vi "Pigeon2Getters.vi"   [LabVIEW 2023]
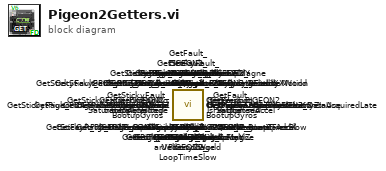
[diagram p0: block diagram]
diagram:
  n1 = call <vilib>:"GetStickyFault_PIGEON2_SaturatedGyros.vi"() -> ()  [unwired: 11 in, 1 out]
  n2 = call <vilib>:"GetFault_PIGEON2_SaturatedGyros.vi"() -> ()  [unwired: 11 in, 1 out]
  n3 = call <vilib>:"GetStickyFault_PIGEON2_SaturatedAccel.vi"() -> ()  [unwired: 11 in, 1 out]
  n4 = call <vilib>:"GetFault_PIGEON2_SaturatedAccel.vi"() -> ()  [unwired: 11 in, 1 out]
  n5 = call <vilib>:"GetStickyFault_PIGEON2_SaturatedMagne.vi"() -> ()  [unwired: 11 in, 1 out]
  n6 = call <vilib>:"GetFault_PIGEON2_SaturatedMagne.vi"() -> ()  [unwired: 11 in, 1 out]
  n7 = call <vilib>:"GetStickyFault_PIGEON2_LoopTimeSlow.vi"() -> ()  [unwired: 11 in, 1 out]
  n8 = call <vilib>:"GetFault_PIGEON2_LoopTimeSlow.vi"() -> ()  [unwired: 11 in, 1 out]
  n9 = call <vilib>:"GetStickyFault_PIGEON2_DataAcquiredLate.vi"() -> ()  [unwired: 11 in, 1 out]
  n10 = call <vilib>:"GetFault_PIGEON2_DataAcquiredLate.vi"() -> ()  [unwired: 11 in, 1 out]
  n11 = call <vilib>:"GetStickyFault_PIGEON2_BootIntoMotion.vi"() -> ()  [unwired: 11 in, 1 out]
  n12 = call <vilib>:"GetFault_PIGEON2_BootIntoMotion.vi"() -> ()  [unwired: 11 in, 1 out]
  n13 = call <vilib>:"GetStickyFault_PIGEON2_BootupMagne.vi"() -> ()  [unwired: 11 in, 1 out]
  n14 = call <vilib>:"GetFault_PIGEON2_BootupMagne.vi"() -> ()  [unwired: 11 in, 1 out]
  n15 = call <vilib>:"GetStickyFault_PIGEON2_BootupGyros.vi"() -> ()  [unwired: 11 in, 1 out]
  n16 = call <vilib>:"GetFault_PIGEON2_BootupGyros.vi"() -> ()  [unwired: 11 in, 1 out]
  n17 = call <vilib>:"GetStickyFault_PIGEON2_BootupAccel.vi"() -> ()  [unwired: 11 in, 1 out]
  n18 = call <vilib>:"GetFault_PIGEON2_BootupAccel.vi"() -> ()  [unwired: 11 in, 1 out]
  n19 = call <vilib>:"GetStickyFault_UnlicensedFeatureInUse.vi"() -> ()  [unwired: 11 in, 1 out]
  n20 = call <vilib>:"GetFault_UnlicensedFeatureInUse.vi"() -> ()  [unwired: 11 in, 1 out]
  n21 = call <vilib>:"GetStickyFault_BootDuringEnable.vi"() -> ()  [unwired: 11 in, 1 out]
  n22 = call <vilib>:"GetFault_BootDuringEnable.vi"() -> ()  [unwired: 11 in, 1 out]
  n23 = call <vilib>:"GetStickyFault_Undervoltage.vi"() -> ()  [unwired: 11 in, 1 out]
  n24 = call <vilib>:"GetFault_Undervoltage.vi"() -> ()  [unwired: 11 in, 1 out]
  n25 = call <vilib>:"GetStickyFault_Hardware.vi"() -> ()  [unwired: 11 in, 1 out]
  n26 = call <vilib>:"GetFault_Hardware.vi"() -> ()  [unwired: 11 in, 1 out]
  n27 = call <vilib>:"GetVersion_IsProLicensed.vi"() -> ()  [unwired: 11 in, 1 out]
  n28 = call <vilib>:"GetPigeon2RawMagneticFieldZ.vi"() -> ()  [unwired: 11 in, 1 out]
  n29 = call <vilib>:"GetPigeon2RawMagneticFieldY.vi"() -> ()  [unwired: 11 in, 1 out]
  n30 = call <vilib>:"GetPigeon2RawMagneticFieldX.vi"() -> ()  [unwired: 11 in, 1 out]
  n31 = call <vilib>:"GetPigeon2MagneticFieldZ.vi"() -> ()  [unwired: 11 in, 1 out]
  n32 = call <vilib>:"GetPigeon2MagneticFieldY.vi"() -> ()  [unwired: 11 in, 1 out]
  n33 = call <vilib>:"GetPigeon2MagneticFieldX.vi"() -> ()  [unwired: 11 in, 1 out]
  n34 = call <vilib>:"GetPigeon2AngularVelocityZ.vi"() -> ()  [unwired: 11 in, 1 out]
  n35 = call <vilib>:"GetPigeon2AngularVelocityY.vi"() -> ()  [unwired: 11 in, 1 out]
  n36 = call <vilib>:"GetPigeon2AngularVelocityX.vi"() -> ()  [unwired: 11 in, 1 out]
  n37 = call <vilib>:"GetPigeon2_SupplyVoltage.vi"() -> ()  [unwired: 11 in, 1 out]
  n38 = call <vilib>:"GetPigeon2AccelerationZ.vi"() -> ()  [unwired: 11 in, 1 out]
  n39 = call <vilib>:"GetPigeon2AccelerationY.vi"() -> ()  [unwired: 11 in, 1 out]
  n40 = call <vilib>:"GetPigeon2AccelerationX.vi"() -> ()  [unwired: 11 in, 1 out]
  n41 = call <vilib>:"GetPigeon2AngularVelocityZWorld.vi"() -> ()  [unwired: 11 in, 1 out]
  n42 = call <vilib>:"GetPigeon2AngularVelocityYWorld.vi"() -> ()  [unwired: 11 in, 1 out]
  n43 = call <vilib>:"GetPigeon2AngularVelocityXWorld.vi"() -> ()  [unwired: 11 in, 1 out]
  n44 = call <vilib>:"GetPigeon2AccumGyroZ.vi"() -> ()  [unwired: 11 in, 1 out]
  n45 = call <vilib>:"GetPigeon2AccumGyroY.vi"() -> ()  [unwired: 11 in, 1 out]
  n46 = call <vilib>:"GetPigeon2AccumGyroX.vi"() -> ()  [unwired: 11 in, 1 out]
  n47 = call <vilib>:"GetPigeon2UpTime.vi"() -> ()  [unwired: 11 in, 1 out]
  n48 = call <vilib>:"GetPigeon2TempCompDisabled.vi"() -> ()  [unwired: 11 in, 1 out]
  n49 = call <vilib>:"GetPigeon2NoMotionCount.vi"() -> ()  [unwired: 11 in, 1 out]
  n50 = call <vilib>:"GetPigeon2NoMotionCalEnabled.vi"() -> ()  [unwired: 11 in, 1 out]
  n51 = call <vilib>:"GetPigeon2Temperature.vi"() -> ()  [unwired: 11 in, 1 out]
  n52 = call <vilib>:"GetPigeon2GravityVectorZ.vi"() -> ()  [unwired: 11 in, 1 out]
  n53 = call <vilib>:"GetPigeon2GravityVectorY.vi"() -> ()  [unwired: 11 in, 1 out]
  n54 = call <vilib>:"GetPigeon2GravityVectorX.vi"() -> ()  [unwired: 11 in, 1 out]
  n55 = call <vilib>:"GetPigeon2QuatZ.vi"() -> ()  [unwired: 11 in, 1 out]
  n56 = call <vilib>:"GetPigeon2QuatY.vi"() -> ()  [unwired: 11 in, 1 out]
  n57 = call <vilib>:"GetPigeon2QuatX.vi"() -> ()  [unwired: 11 in, 1 out]
  n58 = call <vilib>:"GetPigeon2QuatW.vi"() -> ()  [unwired: 11 in, 1 out]
  n59 = call <vilib>:"GetPigeon2Roll.vi"() -> ()  [unwired: 11 in, 1 out]
  n60 = call <vilib>:"GetPigeon2Pitch.vi"() -> ()  [unwired: 11 in, 1 out]
  n61 = call <vilib>:"GetPigeon2Yaw.vi"() -> ()  [unwired: 11 in, 1 out]
  n62 = call <vilib>:"GetAllStickyFaults.vi"() -> ()  [unwired: 11 in, 1 out]
  n63 = call <vilib>:"GetAllFaults.vi"() -> ()  [unwired: 11 in, 1 out]
  n64 = call <vilib>:"GetVersion_Full.vi"() -> ()  [unwired: 11 in, 1 out]
  n65 = call <vilib>:"GetVersion_Build.vi"() -> ()  [unwired: 11 in, 1 out]
  n66 = call <vilib>:"GetVersion_Bugfix.vi"() -> ()  [unwired: 11 in, 1 out]
  n67 = call <vilib>:"GetVersion_Minor.vi"() -> ()  [unwired: 11 in, 1 out]
  n68 = call <vilib>:"GetVersion_Major.vi"() -> ()  [unwired: 11 in, 1 out]
